vi "RunExceldispatchWith2Min.vi"() -> ()   [LabVIEW 2012]
uses:
  <vilib>/Utility/NIReport.llb/NI_report.lvclass
  Global1.vi
  <vilib>/addons/database/Connection.llb/DB Tools Open Connec (Path).vi
  <vilib>/addons/_office/excel.llb/Excel Get Data (str).vi
  <vilib>/Utility/NIReport.llb/Excel/NI_Excel.lvclass
  <vilib>/addons/_office/NI_ReportGenerationToolkit.lvlib
  <vilib>/addons/database/NI_Database_API.lvlib
panel:
  out "error out":errorcluster
  out "error out 4":errorcluster
  out "String 2":string
  out "error out 3":errorcluster
  in  "start (0, 0)":cluster{"start row":i32, "start column":i32}
  out "x+y":i32
  out "row":i32
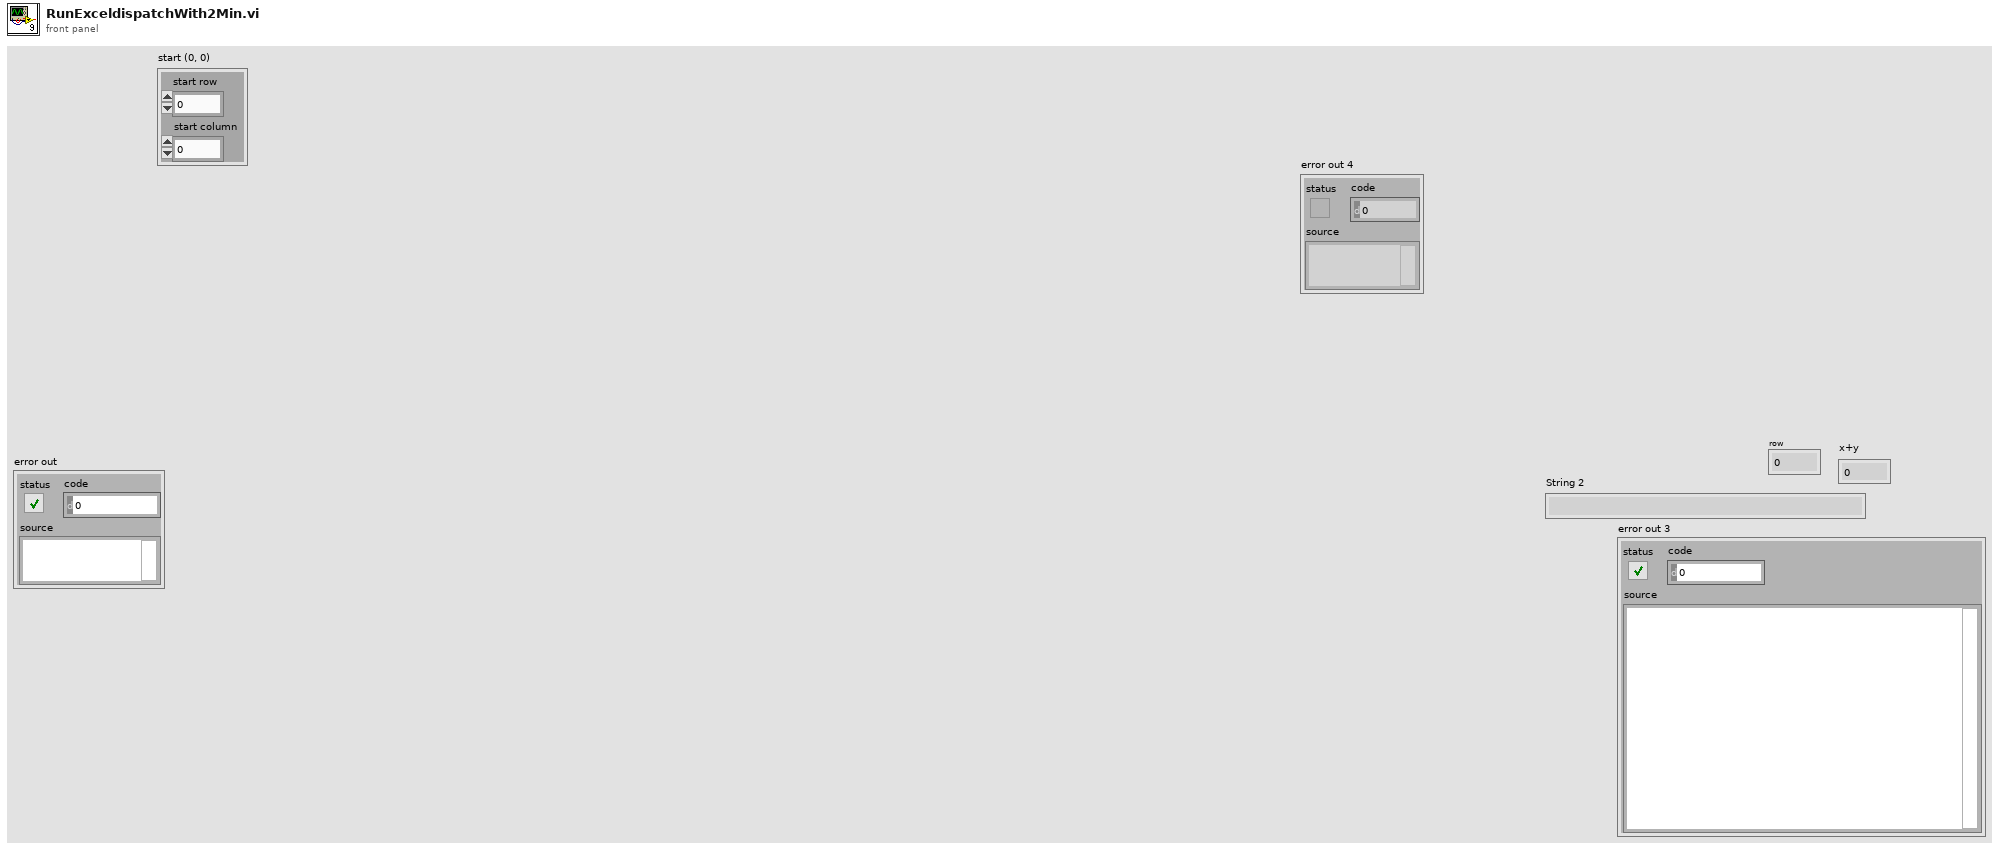
[diagram p1: front panel]
types:
  T1 = enum16{"Standard Report", "HTML", "Word", "Excel"}
  T2 = typedef "NI_Database_API.lvlib/Conn ObjectReference.ctl" = refnum<k1>
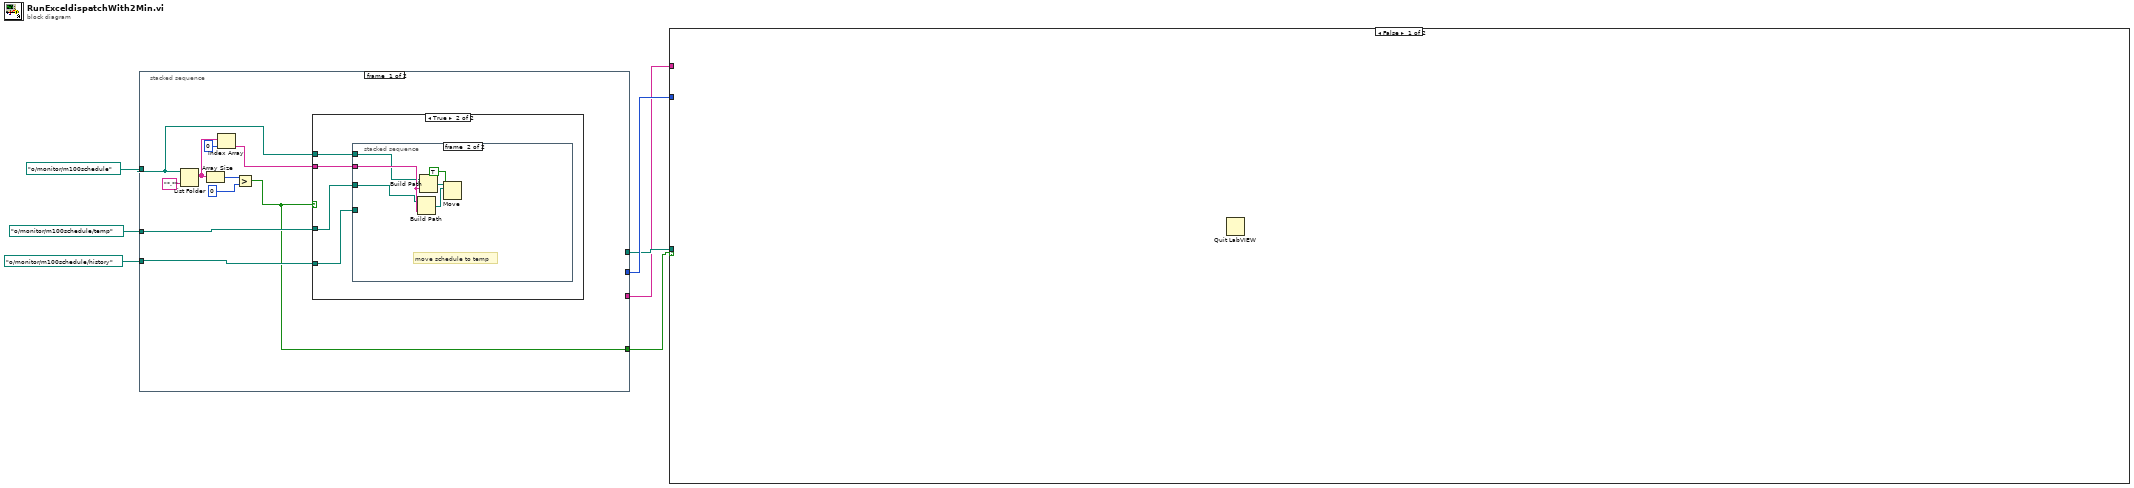
[diagram p0: block diagram]
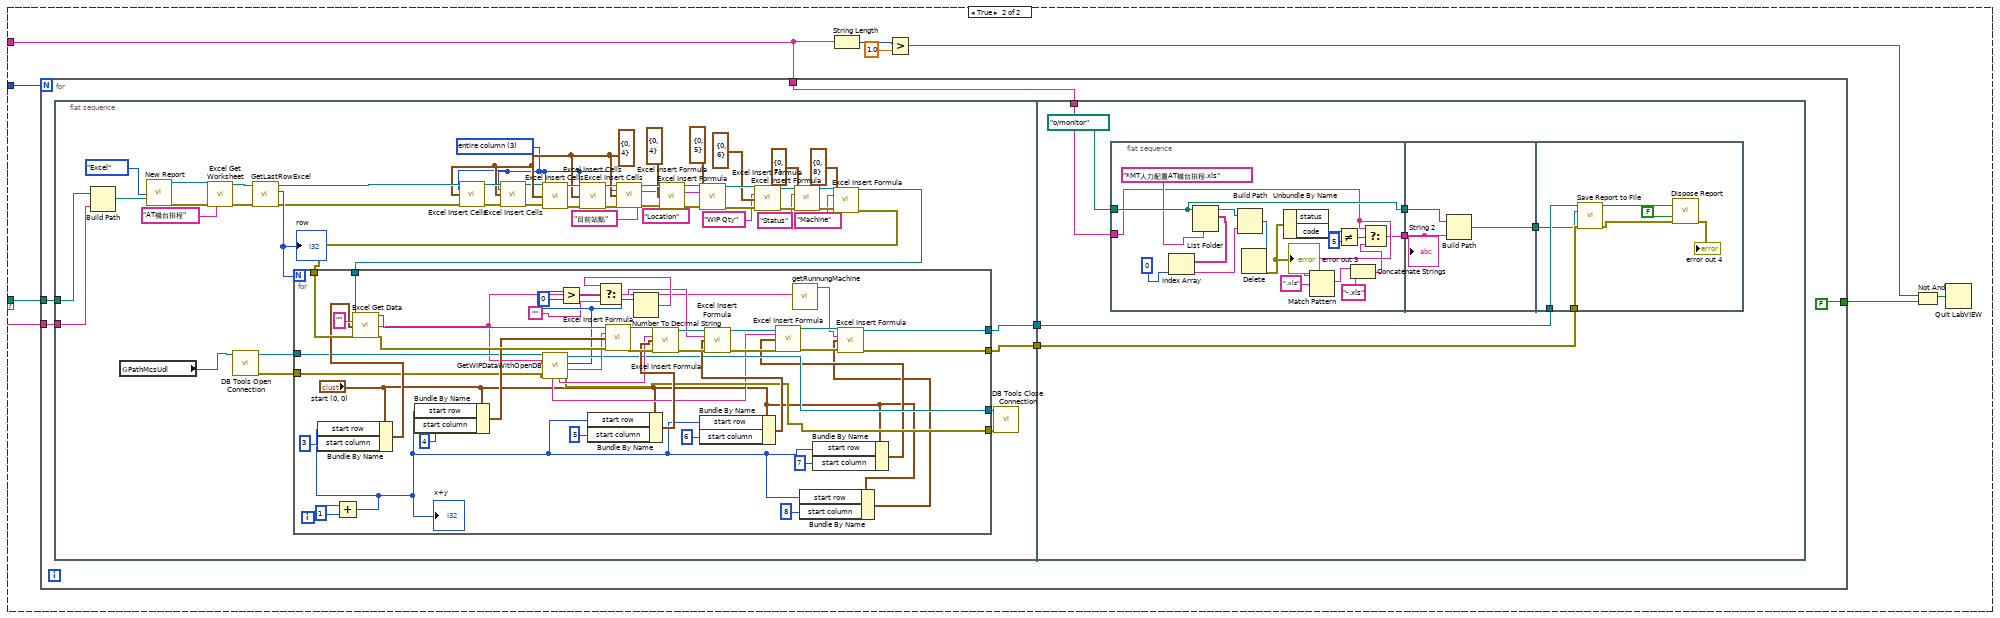
[diagram p2: hidden frame]
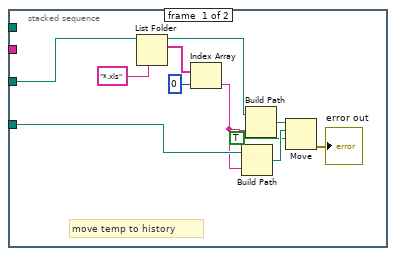
[diagram p4: hidden frame]
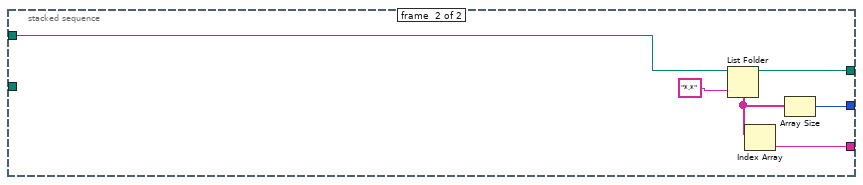
[diagram p5: hidden frame]
diagram:
  n1 = stacked-sequence {
    tunnel: path "o:/monitor/m100schedule/temp" ("path") -> [w9 w43]
    tunnel: [_ w42] -> w6
    tunnel: [_ w41] -> w5
    tunnel: [_ w39] -> w4
    tunnel: path "o:/monitor/m100schedule" ("path") -> [w11 _]
    tunnel: path "o:/monitor/m100schedule/history" ("path") -> [w10 _]
    tunnel: [w8 _] -> w1
    frame #0 {
      n2 = List Folder(path=w11, pattern="*.*") -> (filenames=w14:string[])  [unwired: 2 in, 3 out]
      n3 = Array Size(array=w14) -> (size(s)=w16:i32)
      n4 = Index Array(array=w14, index=0) -> (element=w13:string)
      n5 = Greater?(x=w16, y=0) -> (0:w8:bool)
      n6 = case shown="True" w8 {
        tunnel: w9 -> [_ w21]
        tunnel: w10 -> [_ w20]
        tunnel: w11 -> [_ w19]
        tunnel: w13 -> [_ w18]
        frame False {
        }
        frame True {
          n7 = stacked-sequence {
            tunnel: w21 -> [w28 w34]
            tunnel: w20 -> [w31 _]
            tunnel: w19 -> [_ w35]
            tunnel: w18 -> [_ w36]
            frame #0 {
              # "move temp to history"
              n8 = List Folder(path=w28, pattern="*.xls") -> (path out=w26:path, filenames=w25:string[])  [unwired: 2 in, 2 out]
              n9 = Index Array(array=w25, index=0) -> (element=w23:string)
              n10 = Build Path(base path=w31, name or relative path=w23) -> (appended path=w30:path)
              n11 = Build Path(base path=w26, name or relative path=w23) -> (appended path=w32:path)
              n12 = Move(source path=w32, 9:TRUE ("overwrite (F)"), 10:w30) -> (error out=→"error out":errorcluster)  [unwired: 2 in, 2 out]
            }
            frame #1 {
              # "move schedule to temp"
              n13 = Build Path(base path=w34, name or relative path=w36) -> (appended path=w37:path)
              n14 = Build Path(base path=w35, name or relative path=w36) -> (appended path=w38:path)
              n15 = Move(source path=w38, 9:TRUE ("overwrite (F)"), 10:w37) -> ()  [unwired: 2 in, 3 out]
            }
          }
        }
      }
    }
    frame #1 {
      n16 = List Folder(path=w43, pattern="*.*") -> (path out=w41:path, filenames=w40:string[])  [unwired: 2 in, 2 out]
      n17 = Index Array(array=w40) -> (element=w39:string)  [unwired: 1 in]
      n18 = Array Size(array=w40) -> (size(s)=w42:i32)
    }
  }
  n19 = case shown="False" w1 {
    tunnel: w6 -> [_ w52]
    tunnel: w5 -> [_ w51]
    tunnel: w4 -> [_ w48]
    frame False {
      n20 = Quit LabVIEW() -> ()  [unwired: 1 in]
    }
    frame True {
      n21 = for {
        N: w52 -> [_]
        tunnel: w51 -> [w58]
        tunnel: w48 -> [w57]
        tunnel: w48 -> [w54]
        tunnel: [FALSE] -> w45
        n22 = flat-sequence {
          tunnel: w58 -> [w109]
          tunnel: w57 -> [w108]
          tunnel: [w82] -> w56
          tunnel: [w62] -> w55
          tunnel: w56 -> [w157]
          tunnel: w55 -> [w158]
          tunnel: w54 -> [w159]
          frame #0 {
            w74 = cluster{"row":i32, "column":i32} {"row"=0, "column"=4} ("start (0, 0)")
            w71 = u16 3 items=["shift cells right", "shift cells down", "entire row", "entire column"] ("mode (entire row)")
            n23 = Build Path(base path=w109, name or relative path=w108) -> (appended path=w107:path)
            n24 = global read "Global1.vi" "PathMcsUdl"() -> (w97:path)
            n25 = call <vilib>:"New Report.vi"("report type"=T1."Excel" ("Report Type"), "template (empty)"=w107) -> ("report out"=w105:refnum<class "NI_report.lvclass">, "error out"=w104:errorcluster)  [unwired: 12 in]
            n26 = call <vilib>:"Excel Get Worksheet.vi"("report in"=w105, "error in (no error)"=w104, "name (\"\")"="AT機台排程" ("name (\"\")")) -> ("report out"=w81:refnum<class "NI_report.lvclass">, "error out"=w80:errorcluster)  [unwired: 11 in]
            n27 = call-poly <vilib>:"DB Tools Open Connection.vi"("connection information"=w97) -> ("error out"=w95:errorcluster, "connection reference"=w96:T2)  [unwired: 7 in]
            n28 = call "GetLastRowExcel.vi"("error in (no error)"=w80, "report in"=w81) -> ("error out"=w78:errorcluster, "row"=w79:i32, "report out"=w77:refnum<class "NI_report.lvclass">)  [unwired: 7 in]
            "row" <- w79
            n29 = call <vilib>:"Excel Insert Cells.vi"("report in"=w77, "mode (entire row)"=w71, "start (0, 0)"=w74, "error in (no error)"=w78) -> ("report out"=w76:refnum<class "NI_report.lvclass">, "error out"=w75:errorcluster)  [unwired: 10 in]
            n30 = call <vilib>:"Excel Insert Cells.vi"("report in"=w76, "mode (entire row)"=w71, "start (0, 0)"=w74, "error in (no error)"=w75) -> ("report out"=w73:refnum<class "NI_report.lvclass">, "error out"=w72:errorcluster)  [unwired: 10 in]
            n31 = call <vilib>:"Excel Insert Cells.vi"("report in"=w73, "mode (entire row)"=w71, "start (0, 0)"=w74, "error in (no error)"=w72) -> ("report out"=w103:refnum<class "NI_report.lvclass">, "error out"=w101:errorcluster)  [unwired: 10 in]
            n32 = call <vilib>:"Excel Insert Cells.vi"("report in"=w103, "mode (entire row)"=w71, "start (0, 0)"=w74, "error in (no error)"=w101) -> ("report out"=w102:refnum<class "NI_report.lvclass">, "error out"=w100:errorcluster)  [unwired: 10 in]
            n33 = call <vilib>:"Excel Insert Cells.vi"("report in"=w102, "mode (entire row)"=w71, "start (0, 0)"=w74, "error in (no error)"=w100) -> ("report out"=w94:refnum<class "NI_report.lvclass">, "error out"=w91:errorcluster)  [unwired: 10 in]
            n34 = call <vilib>:"Excel Insert Formula.vi"("report in"=w94, "formula"="目前站點", "start (0, 0)"=cluster{"row":i32, "column":i32} {"row"=0, "column"=4}, "error in (no error)"=w91) -> ("report out"=w93:refnum<class "NI_report.lvclass">, "error out"=w90:errorcluster)  [unwired: 10 in]
            n35 = call <vilib>:"Excel Insert Formula.vi"("report in"=w93, "formula"="Location", "start (0, 0)"=cluster{"row":i32, "column":i32} {"row"=0, "column"=5}, "error in (no error)"=w90) -> ("report out"=w92:refnum<class "NI_report.lvclass">, "error out"=w89:errorcluster)  [unwired: 10 in]
            n36 = call <vilib>:"Excel Insert Formula.vi"("report in"=w92, "formula"="WIP Qty", "start (0, 0)"=cluster{"row":i32, "column":i32} {"row"=0, "column"=6}, "error in (no error)"=w89) -> ("report out"=w70:refnum<class "NI_report.lvclass">, "error out"=w68:errorcluster)  [unwired: 10 in]
            n37 = call <vilib>:"Excel Insert Formula.vi"("report in"=w70, "formula"="Status", "start (0, 0)"=cluster{"row":i32, "column":i32} {"row"=0, "column"=7}, "error in (no error)"=w68) -> ("report out"=w69:refnum<class "NI_report.lvclass">, "error out"=w67:errorcluster)  [unwired: 10 in]
            n38 = call <vilib>:"Excel Insert Formula.vi"("report in"=w69, "formula"="Machine", "start (0, 0)"=cluster{"row":i32, "column":i32} {"row"=0, "column"=8}, "error in (no error)"=w67) -> ("report out"=w65:refnum<class "NI_report.lvclass">, "error out"=w66:errorcluster)  [unwired: 10 in]
            n39 = for {
              N: w79 -> [_]
              tunnel: w65 -> [w155]
              tunnel: w66 -> [w154]
              tunnel: [w118] -> w82
              tunnel: [w136] -> w99
              tunnel: [w135] -> w98
              tunnel: w96 -> [w134]
              tunnel: w95 -> [w133]
              tunnel: [w119] -> w62
              i -> [w126]
              n40 = Add(x=w126, y=1) -> (x+y=w115:i32)
              "x+y" <- w115
              n41 = Bundle By Name(cluster="start (0, 0)", "start row"=w115, "start column"=3) -> (w149:cluster{"start row":i32, "start column":i32})
              n42 = call-poly <vilib>:"Excel Get Data.vi"("report in"=w155, "data type"="", "start (0, 0)"=w149, "error in (no error)"=w154) -> ("report out"=w152:refnum<class "NI_report.lvclass">, "data"=w110:string, "error out"=w151:errorcluster)  [unwired: 9 in]
              n43 = Bundle By Name(cluster="start (0, 0)", "start row"=w115, "start column"=4) -> (w147:cluster{"start row":i32, "start column":i32})
              n44 = call "GetWIPDataWithOpenDB.vi"("error in (no error)"=w133, "Lotno"=w110, "connection reference"=w134) -> ("error out"=w135:errorcluster, "step"=w138:string, "data"=w131:i32, "connection reference 2"=w136:T2, "location"=w137:string, "status"=w116:string)  [unwired: 3 in]
              n45 = Greater?(x=w131, y=0) -> (0:w129:bool)
              n46 = Bundle By Name(cluster="start (0, 0)", "start row"=w115, "start column"=5) -> (w139:cluster{"start row":i32, "start column":i32})
              n47 = call <vilib>:"Excel Insert Formula.vi"("report in"=w152, "formula"=w138, "start (0, 0)"=w147, "error in (no error)"=w151) -> ("report out"=w144:refnum<class "NI_report.lvclass">, "error out"=w141:errorcluster)  [unwired: 10 in]
              n48 = Number To Decimal String(number=w131) -> (decimal integer string=w130:string)  [unwired: 1 in]
              n49 = Select(t=w130, s=w129, f="") -> (s? t:f=w127:string)
              n50 = call <vilib>:"Excel Insert Formula.vi"("report in"=w144, "formula"=w137, "start (0, 0)"=w139, "error in (no error)"=w141) -> ("report out"=w143:refnum<class "NI_report.lvclass">, "error out"=w142:errorcluster)  [unwired: 10 in]
              n51 = Bundle By Name(cluster="start (0, 0)", "start row"=w115, "start column"=6) -> (w140:cluster{"start row":i32, "start column":i32})
              n52 = call <vilib>:"Excel Insert Formula.vi"("report in"=w143, "formula"=w127, "start (0, 0)"=w140, "error in (no error)"=w142) -> ("report out"=w123:refnum<class "NI_report.lvclass">, "error out"=w122:errorcluster)  [unwired: 10 in]
              n53 = call "getRunnungMachine.vi"("rc_no"=w110) -> ("machine"=w111:string)  [unwired: 9 in, 1 out]
              n54 = Bundle By Name(cluster="start (0, 0)", "start row"=w115, "start column"=8) -> (w113:cluster{"start row":i32, "start column":i32})
              n55 = Bundle By Name(cluster="start (0, 0)", "start row"=w115, "start column"=7) -> (w117:cluster{"start row":i32, "start column":i32})
              n56 = call <vilib>:"Excel Insert Formula.vi"("report in"=w123, "formula"=w116, "start (0, 0)"=w117, "error in (no error)"=w122) -> ("report out"=w121:refnum<class "NI_report.lvclass">, "error out"=w120:errorcluster)  [unwired: 10 in]
              n57 = call <vilib>:"Excel Insert Formula.vi"("report in"=w121, "formula"=w111, "start (0, 0)"=w113, "error in (no error)"=w120) -> ("report out"=w119:refnum<class "NI_report.lvclass">, "error out"=w118:errorcluster)  [unwired: 10 in]
            }
            n58 = call <vilib>:"DB Tools Close Connection.vi"("error in (no error)"=w98, "connection reference"=w99) -> ()  [unwired: 5 in, 1 out]
          }
          frame #1 {
            n59 = flat-sequence {
              tunnel: path "o:/monitor" ("base path") -> [w175]
              tunnel: [w175] -> w162
              tunnel: w159 -> [w168]
              tunnel: [w163] -> w161
              tunnel: w162 -> [w182]
              tunnel: w161 -> [w181]
              tunnel: [w180] -> w156
              tunnel: w158 -> [w185]
              tunnel: w157 -> [w184]
              tunnel: w156 -> [w183]
              frame #0 {
                n60 = List Folder(path=w175, pattern="*MT人力配置AT機台排程.xls") -> (path out=w177:path, filenames=w179:string[])  [unwired: 2 in, 2 out]
                n61 = Index Array(array=w179, index=0) -> (element=w176:string)
                n62 = Build Path(base path=w177, name or relative path=w176) -> (appended path=w173:path)
                n63 = Delete(path (use dialog)=w173) -> (error out=w172:errorcluster)  [unwired: 4 in, 2 out]
                "error out 3" <- w172
                n64 = Unbundle By Name(w172) -> ("code"=w171:i32)  [unwired: 1 out]
                n65 = Match Pattern(string=w168, regular expression=".xls") -> (match substring=w165:string)  [unwired: 1 in, 3 out]
                n66 = Not Equal?(x=w171, y=5) -> (x != y?=w169:bool)
                n67 = Concatenate Strings(w165, "-.xls" ("string")) -> (w166:string)
                n68 = Select(t=w168, s=w169, f=w166) -> (s? t:f=w163:string)
              }
              frame #1 {
                n69 = Build Path(base path=w182, name or relative path=w181) -> (appended path=w180:path)
                "String 2" <- w181
              }
              frame #2 {
                n70 = call-dynamic "Save Report to File.vi"("report in"=w185, "report file path"=w183, "error in (no error)"=w184) -> ("report out"=w186:refnum<class "NI_report.lvclass">, "error out"=w187:errorcluster)  [unwired: 11 in]
                n71 = call-dynamic "Dispose Report.vi"("report in"=w186, "save changes? (F)"=FALSE, "error in (no error)"=w187) -> ("error out"=→"error out 4":errorcluster)  [unwired: 12 in]
              }
            }
          }
        }
      }
      n72 = String Length(string=w48) -> (length=w49:i32)
      n73 = Greater?(x=w49, y=1.0) -> (0:w46:bool)
      n74 = Not And(1:w45, 2:w46) -> (0:w47:bool)
      n75 = Quit LabVIEW(quit? (T)=w47) -> ()
    }
  }
